vi "mod_Add Phase Noise.vi"(0 "input complex waveform":T3={"t0"=0.0, "dt"=1.0, "Y"=[]} {"Y" format="%.3f"; "dt" format="%^.2e"; "t0" format="%.4f"}, 1 "1/f filter specifications":T1={"lower cutoff freq"=0.0001, "higher cutoff freq (-1 = Nyquist)"=-1.0, "order"=32}, 5 "noise density at reference (dBc/Hz)":dbl=-100.0 format="%.2p", 7 "offset frequency (Hz)":dbl=0.2 format="%.2p", 9 "exponent n for 1/f^n":dbl=2.0 format="%.2p", 11 "error in (no error)":errorcluster, 12 "seed in":i32=-1 format="%.0x", 13 "reset?":bool) -> (4 "output complex waveform":T3 {"Y" format="%.3f"; "dt" format="%^.2e"; "t0" format="%.4f"}, 8 "Expected RMS":dbl, 10 "seed out":i32=-1 format="%.0x", 14 "noise shaping\nfilter info":T2, 15 "error out":errorcluster)   [LabVIEW 2020, in "niDMT.lvlib"]
uses:
  <vilib>/addons/Modulation/niDMT.lvlib
  <vilib>/addons/Modulation/Analog/controls/Complex Data Waveform.ctl
  <vilib>/addons/Modulation/Digital/General/subVIs/mod_Generate Bits PN Sequence.vi
  <vilib>/Analysis/baseanly.llb/Inverse f Filter (DBL).vi
  <vilib>/Analysis/NI_AALPro.lvlib
  <vilib>/Analysis/NI_AALBase.lvlib
  <vilib>/addons/Modulation/niAMT.lvlib
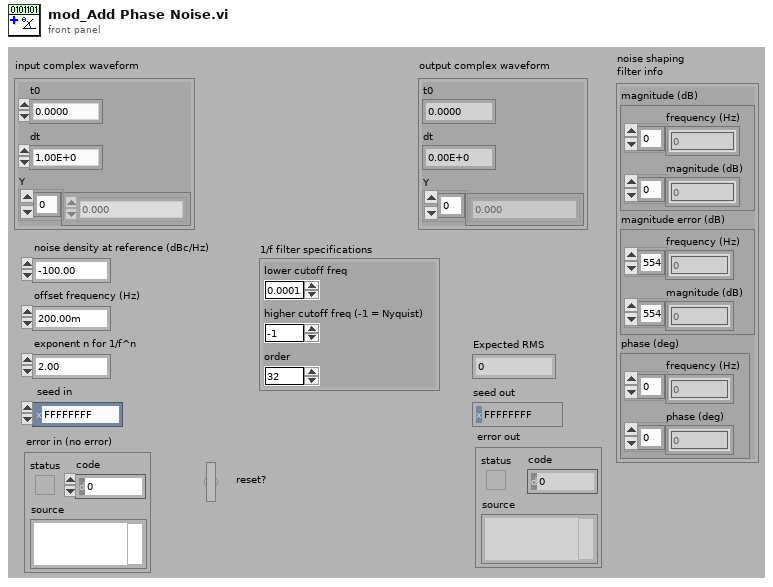
[diagram p1: front panel]
types:
  T1 = cluster{"lower cutoff freq":dbl, "higher cutoff freq (-1 = Nyquist)":dbl, "order":i32}
  T2 = cluster{"magnitude (dB)":cluster{"frequency (Hz)":dbl[], "magnitude (dB)":dbl[]}, "magnitude error (dB)":cluster{"frequency (Hz)":dbl[], "magnitude (dB)":dbl[]}, "phase (deg)":cluster{"frequency (Hz)":dbl[], "phase (deg)":dbl[]}}
  T3 = typedef "niAMT.lvlib/Complex Data Waveform.ctl" = cluster{"t0":dbl, "dt":dbl, "Y":cdb[]}
  T4 = cluster{"frequency (Hz)":dbl[], "magnitude (dB)":dbl[]}
  T5 = cluster{"magnitude (dB)":cluster{"frequency (Hz)":dbl[], "magnitude (dB)":dbl[]}, "phase (deg)":cluster{"frequency (Hz)":dbl[], "phase (deg)":dbl[]}}
  T6 = cluster{"frequency (Hz)":dbl[], "phase (deg)":dbl[]}
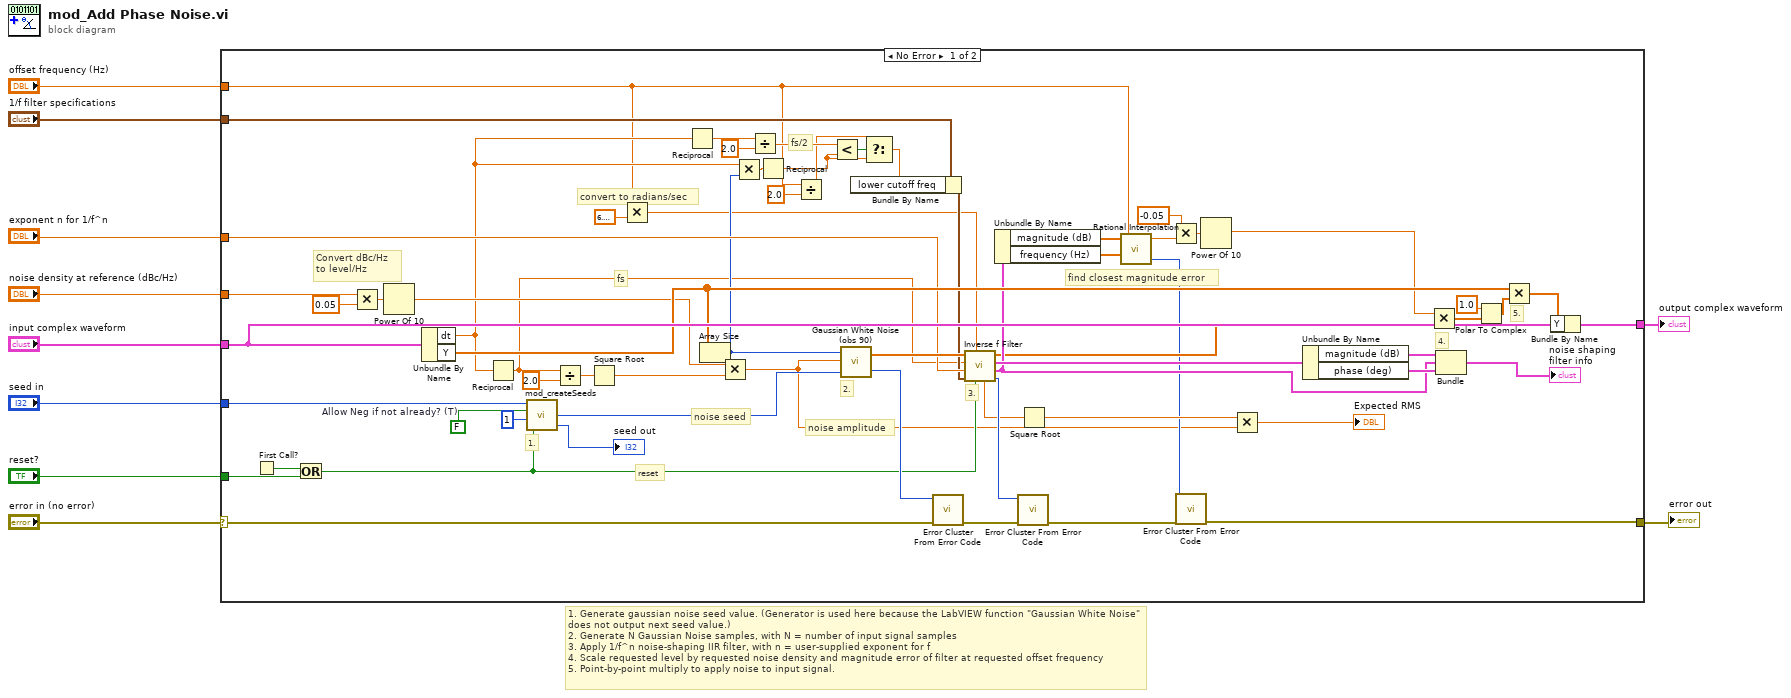
[diagram p0: block diagram]
diagram:
  # "1. Generate gaussian noise seed value. (Generator is used here because the LabVIEW function \"Gaussian White Noise\" does not output next seed value.)\n2. Generate N Gaussian Noise samples, with N = number of input signal samples\n3. Apply 1/f^n noise-shaping IIR filter, with n = user-supplied exponent for f\n4. Scale requested level by requested noise density and magnitude error of filter at requested offset frequency \n5. Point-by-point multiply to apply noise to input signal."
  n1 = case shown="No Error" "error in (no error)" {
    selector: "error in (no error)" -> [w53 w75]
    tunnel: "input complex waveform" -> [w74 w76]
    tunnel: "noise density at reference (dBc/Hz)" -> [w73 _]
    tunnel: "seed in" -> [w72 _]
    tunnel: "reset?" -> [w45 _]
    tunnel: "exponent n for 1/f^n" -> [w52 _]
    tunnel: "offset frequency (Hz)" -> [w14 _]
    tunnel: [w54 w76] -> w4
    tunnel: [w29 w75] -> w3
    tunnel: "1/f filter specifications" -> [w40 _]
    frame No Error {
      w33 = FALSE  # Allow Neg if not already? (T)
      # "fs/2"
      # "find closest magnitude error"
      # "Convert dBc/Hz\nto level/Hz"
      # "convert to radians/sec"
      # "5."
      # "4."
      # "reset"
      # "noise amplitude"
      # "fs"
      # "1."
      # "3."
      # "2."
      # "noise seed"
      n2 = First Call?() -> (First Call?: T/F=w47:bool)
      n3 = Or(x=w47, y=w45) -> (x .or. y?=w46:bool)
      n4 = Multiply(x=w73, y=0.05) -> (x*y=w63:dbl)
      n5 = Power Of 10(x=w63) -> (10^x=w57:dbl)
      n6 = Unbundle By Name(w74) -> ("dt"=w18:dbl, "Y"=w69:cdb[])
      n7 = Reciprocal(x=w18) -> (1/x=w23:dbl)
      n8 = call <vilib>:"mod_createSeeds.vi"("Reset? (T)"=w46, "# of seeds to create"=1, "Allow Neg if not already? (T)"=w33, "seed in (0xFFFFFFFF)"=w72) -> ("Next seed"=→"seed out":i32, "First Seed"=w59:i32)  [unwired: 1 out]
      n9 = Divide(x=w23, y=2.0) -> (x/y=w24:dbl)
      n10 = Square Root(x=w24) -> (sqrt(x)=w36:dbl)
      n11 = Multiply(x=w14, y=6.283185307179586) -> (x*y=w21:dbl)
      n12 = Reciprocal(x=w18) -> (1/x=w19:dbl)
      n13 = Array Size(array=w69) -> (size(s)=w42:i32)
      n14 = Multiply(x=w57, y=w36) -> (x*y=w25:dbl)
      n15 = Multiply(x=w18, y=w42) -> (x*y=w41:dbl)
      n16 = Divide(x=w19, y=2.0) -> (x/y=w15:dbl)
      n17 = Reciprocal(x=w41) -> (1/x=w11:dbl)
      n18 = Divide(x=w14, y=2.0) -> (x/y=w12:dbl)
      n19 = Less?(x=w15, y=w11) -> (x < y?=w17:bool)
      n20 = call <vilib>:"Gaussian White Noise (obs 90).vi"("seed"=w59, "standard deviation"=w25, "samples"=w42) -> ("error"=w67:i32, "Gaussian noise pattern"=w66:dbl[])
      n21 = Select(t=w12, s=w17, f=w11) -> (s? t:f=w16:dbl)
      n22 = Bundle By Name(cluster=w40, "lower cutoff freq"=w16) -> (w39:T1)
      n23 = call <vilib>:"Error Cluster From Error Code.vi"("error in (no error)"=w53, "error code (0)"=w67) -> ("error out"=w65:errorcluster)  [unwired: 1 in, 6 out]
      n24 = call-poly <vilib>:"Inverse f Filter.vi"("unity gain freq (rad/s)"=w21, "reset"=w46, "filter specifications"=w39, "exponent"=w52, "fs"=w23, "X"=w66) -> ("error"=w64:i32, "magnitude error (dB)"=w48:T4, "filter information"=w56:T5, "Filtered X"=w44:dbl[], "noise bandwidth"=w37:dbl)  [unwired: 1 out]
      n25 = Unbundle By Name(w48) -> ("magnitude (dB)"=w32:dbl[], "frequency (Hz)"=w31:dbl[])
      n26 = call <vilib>:"Error Cluster From Error Code.vi"("error in (no error)"=w65, "error code (0)"=w64) -> ("error out"=w30:errorcluster)  [unwired: 1 in, 6 out]
      n27 = Square Root(x=w37) -> (sqrt(x)=w34:dbl)
      n28 = call <vilib>:"Rational Interpolation.vi"("x value"=w14, "X"=w31, "Y"=w32) -> ("error"=w28:i32, "interpolation value"=w27:dbl)  [unwired: 1 out]
      n29 = Multiply(x=-0.05 ("y"), y=w27) -> (x*y=w49:dbl)
      n30 = call <vilib>:"Error Cluster From Error Code.vi"("error in (no error)"=w30, "error code (0)"=w28) -> ("error out"=w29:errorcluster)  [unwired: 1 in, 6 out]
      n31 = Power Of 10(x=w49) -> (10^x=w35:dbl)
      n32 = Multiply(x=w34, y=w25) -> (x*y=→"Expected RMS":dbl)
      n33 = Unbundle By Name(w56) -> ("magnitude (dB)"=w50:T4, "phase (deg)"=w55:T6)
      n34 = Multiply(x=w35, y=w44) -> (x*y=w43:dbl[])
      n35 = Bundle("magnitude (dB)"=w50, "magnitude error (dB)"=w48, "phase (deg)"=w55) -> (→"noise shaping\nfilter info":T2)  [unwired: 1 out]
      n36 = Polar To Complex(1:w43, 2:1.0) -> (0:w70:cdb[])
      n37 = Multiply(x=w69, y=w70) -> (x*y=w68:cdb[])
      n38 = Bundle By Name(cluster=w74, "Y"=w68) -> (w54:T3)
    }
    frame Error {
    }
  }
  "output complex waveform" <- w4
  "error out" <- w3
